vi "Receiver 17 new version.vi"   [LabVIEW 2012]
uses:
  <vilib>/NXT/Block Support/NXT_MessageMailbox.ctl
  <vilib>/NXT/Subs/MotorOutput.ctl
  <vilib>/NXT/Block Support/NXT_InputPort.ctl
  <vilib>/NXT/Dual Mode Library/Waits/Wait_Num.vi
  <vilib>/NXT/Dual Mode Library/BT/BlueTooth_Read_string.vi
  <vilib>/NXT/Dual Mode Library/Display/drawText.vi
types:
  T1 = typedef "LVHSConnector.ctl" = refnum<class "BrickReference.lvclass">
  T2 = typedef "NXT_MessageMailbox.ctl" = u8
  T3 = typedef "MotorOutput.ctl" = u8
  T4 = typedef "NXT_InputPort.ctl" = u32
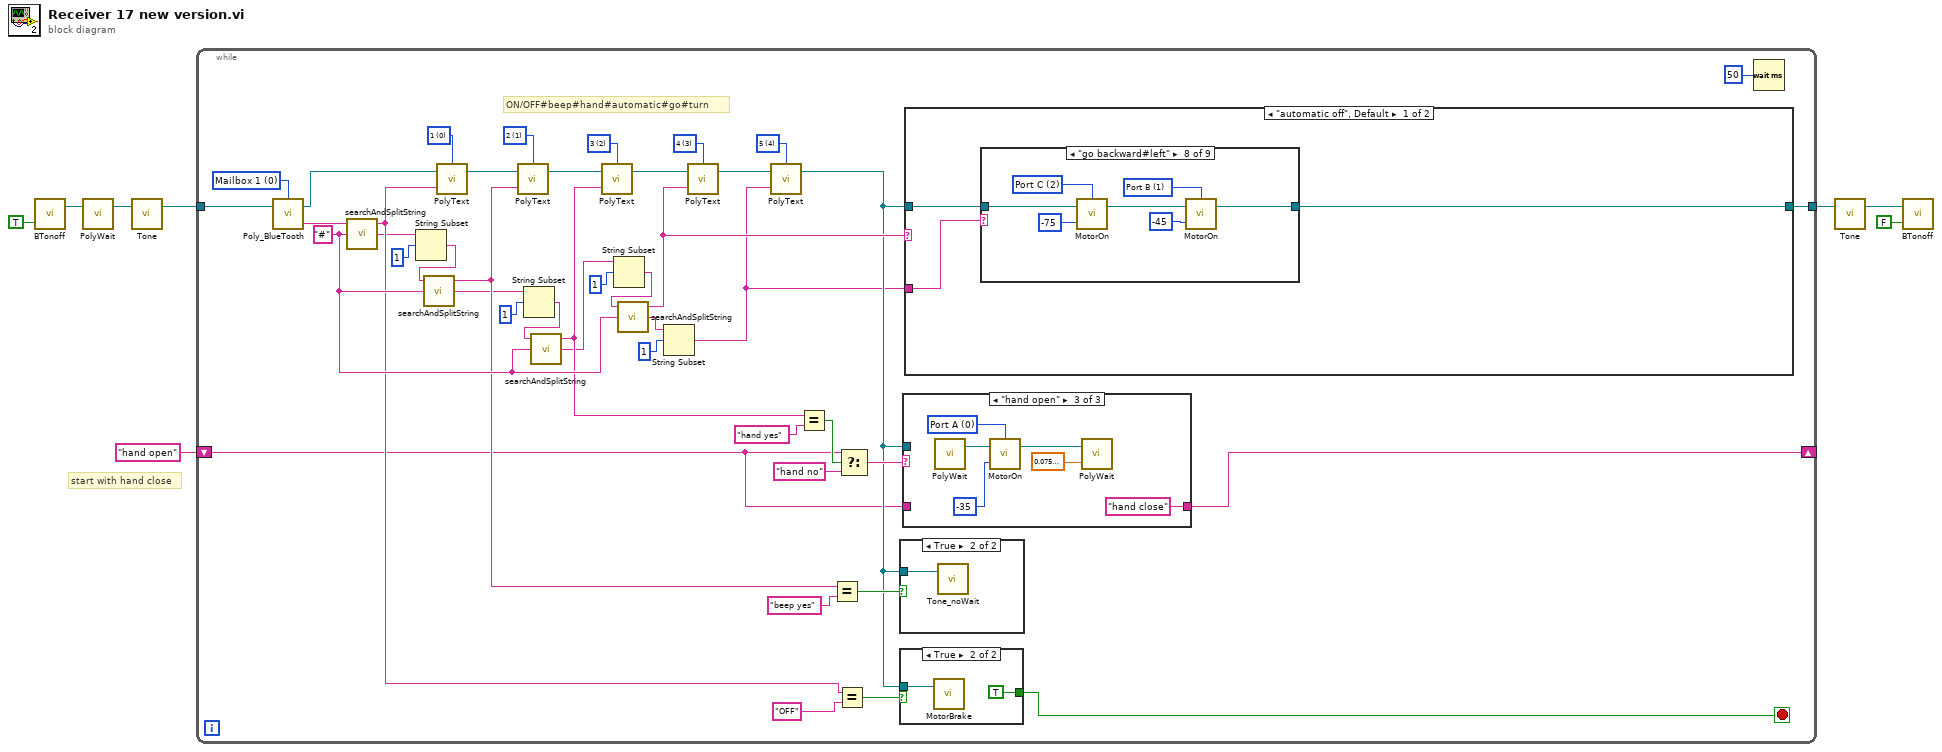
[diagram p0: block diagram]
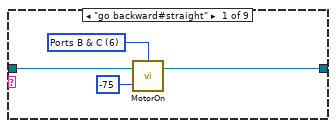
[diagram p2: hidden frame]
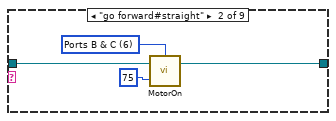
[diagram p3: hidden frame]
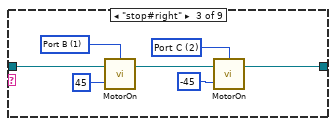
[diagram p4: hidden frame]
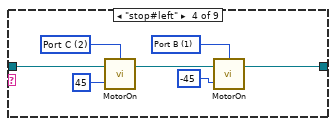
[diagram p5: hidden frame]
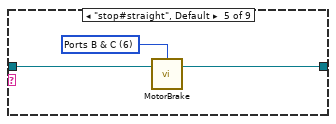
[diagram p6: hidden frame]
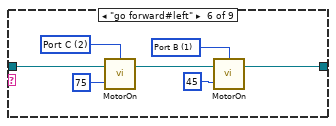
[diagram p7: hidden frame]
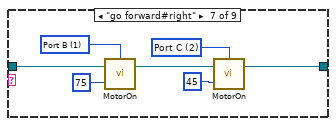
[diagram p8: hidden frame]
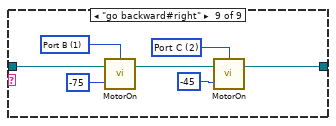
[diagram p9: hidden frame]
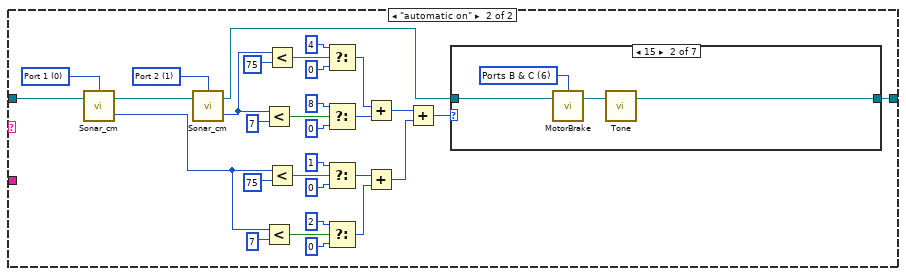
[diagram p10: hidden frame]
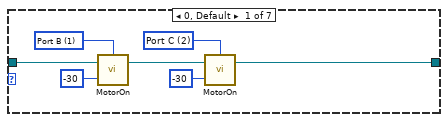
[diagram p11: hidden frame]
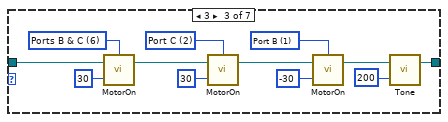
[diagram p12: hidden frame]
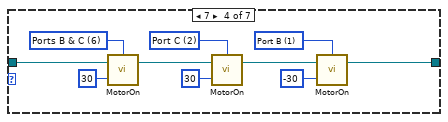
[diagram p13: hidden frame]
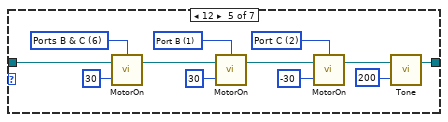
[diagram p14: hidden frame]
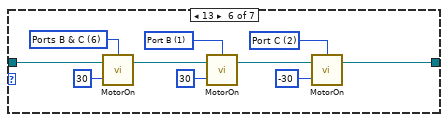
[diagram p15: hidden frame]
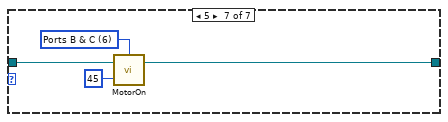
[diagram p16: hidden frame]
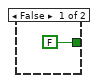
[diagram p17: hidden frame]
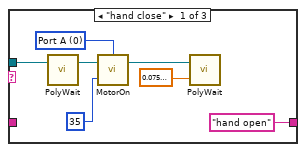
[diagram p19: hidden frame]
diagram:
  # "start with hand close"
  n1 = call <vilib>:"BTonoff.vi"("On/Off"=TRUE) -> ("NXT/EV3"=w6:T1)  [unwired: 2 in, 1 out]
  n2 = call-poly <vilib>:"PolyWait.vi"("NXT/EV3"=w6) -> ("NXT/EV3"=w4:T1)  [unwired: 3 in]
  n3 = call <vilib>:"Tone.vi"("NXT/EV3"=w4) -> ("NXT/EV3"=w3:T1)  [unwired: 3 in]
  n4 = while {
    tunnel: w3 -> [w50]
    shift-right: [w46] -> _
    shift-left: "hand open" -> [w10]
    tunnel: [w41] -> w1
    stop <- w36 stop-if-true
    w28 = i16 4 items=["1", "2", "3", "4", "5", "6", "7", "8", "9", "10", "11", "12"] ("Line")
    w30 = i16 3 items=["1", "2", "3", "4", "5", "6", "7", "8", "9", "10", "11", "12"] ("Line")
    w32 = i16 2 items=["1", "2", "3", "4", "5", "6", "7", "8", "9", "10", "11", "12"] ("Line")
    w34 = i16 1 items=["1", "2", "3", "4", "5", "6", "7", "8", "9", "10", "11", "12"] ("Line")
    w35 = i16 0 items=["1", "2", "3", "4", "5", "6", "7", "8", "9", "10", "11", "12"] ("Line")
    w39 = "#" ("search string/char (-)")
    w52 = T2 0 items=["Mailbox 1", "Mailbox 2", "Mailbox 3", "Mailbox 4", "Mailbox 5", "Mailbox 6", "Mailbox 7", "Mailbox 8", "Mailbox 9", "Mailbox 10"] ("Mailbox")
    # "ON/OFF#beep#hand#automatic#go#turn"
    n5 = call-poly <vilib>:"Poly_BlueTooth.vi"("NXT/EV3"=w50, "Mailbox"=w52) -> ("Message"=w40:string, "NXT/EV3"=w26:T1)  [unwired: 1 in]
    n6 = call <vilib>:"searchAndSplitString.vi"("search string/char (-)"=w39, "string"=w40) -> ("match + rest of string"=w18:string, "substring before match"=w25:string)  [unwired: 1 in, 1 out]
    n7 = String Subset(string=w18, offset (0)=1) -> (substring=w14:string)  [unwired: 1 in]
    n8 = call <vilib>:"searchAndSplitString.vi"("search string/char (-)"=w39, "string"=w14) -> ("match + rest of string"=w16:string, "substring before match"=w24:string)  [unwired: 1 in, 1 out]
    n9 = call-poly <vilib>:"PolyText.vi"("Text"=w25, "NXT/EV3"=w26, "Line"=w35) -> ("NXT/EV3"=w33:T1)  [unwired: 1 in]
    n10 = call-poly <vilib>:"PolyText.vi"("Text"=w24, "NXT/EV3"=w33, "Line"=w34) -> ("NXT/EV3"=w31:T1)  [unwired: 1 in]
    n11 = String Subset(string=w16, offset (0)=1) -> (substring=w15:string)  [unwired: 1 in]
    n12 = call <vilib>:"searchAndSplitString.vi"("search string/char (-)"=w39, "string"=w15) -> ("match + rest of string"=w12:string, "substring before match"=w23:string)  [unwired: 1 in, 1 out]
    n13 = call-poly <vilib>:"PolyText.vi"("Text"=w23, "NXT/EV3"=w31, "Line"=w32) -> ("NXT/EV3"=w29:T1)  [unwired: 1 in]
    n14 = String Subset(string=w12, offset (0)=1) -> (substring=w11:string)  [unwired: 1 in]
    n15 = call <vilib>:"searchAndSplitString.vi"("search string/char (-)"=w39, "string"=w11) -> ("match + rest of string"=w37:string, "substring before match"=w22:string)  [unwired: 1 in, 1 out]
    n16 = String Subset(string=w37, offset (0)=1) -> (substring=w20:string)  [unwired: 1 in]
    n17 = call-poly <vilib>:"PolyText.vi"("Text"=w22, "NXT/EV3"=w29, "Line"=w30) -> ("NXT/EV3"=w27:T1)  [unwired: 1 in]
    n18 = call-poly <vilib>:"PolyText.vi"("Text"=w20, "NXT/EV3"=w27, "Line"=w28) -> ("NXT/EV3"=w21:T1)  [unwired: 1 in]
    n19 = Equal?(x=w23, y="hand yes") -> (x = y?=w48:bool)
    n20 = Equal?(x=w24, y="beep yes") -> (x = y?=w44:bool)
    n21 = Equal?(x=w25, y="OFF") -> (x = y?=w42:bool)
    n22 = Select(t=w10, s=w48, f="hand no") -> (s? t:f=w47:string)
    n23 = case shown="True" w44 {
      tunnel: w21 -> [_ w202]
      frame False {
      }
      frame True {
        n24 = call <vilib>:"Tone_noWait.vi"("NXT/EV3"=w202) -> ()  [unwired: 3 in, 1 out]
      }
    }
    n25 = case shown="True" w42 {
      tunnel: [FALSE TRUE] -> w36
      tunnel: w21 -> [_ w200]
      frame False {
      }
      frame True {
        n26 = call <vilib>:"MotorBrake.vi"("NXT/EV3"=w200) -> ()  [unwired: 3 in, 1 out]
      }
    }
    n27 = case shown="\"hand open\"" w47 {
      tunnel: ["hand open" w210 "hand close"] -> w46
      tunnel: w21 -> [w203 _ _]
      tunnel: w10 -> [_ w210 _]
      frame "hand close" {
        w209 = T3 0 items=["Port A"=0, "Port B"=1, "Port C"=2, "Ports A & B"=4, "Ports A & C"=5, "Ports B & C"=6, "All Ports"=3] ("Output Port (All Ports)")
        n28 = call-poly <vilib>:"PolyWait.vi"("NXT/EV3"=w203) -> ("NXT/EV3"=w205:T1)  [unwired: 3 in]
        n29 = call <vilib>:"MotorOn.vi"("Power (75)"=35, "NXT/EV3"=w205, "Output Port (All Ports)"=w209) -> ("NXT/EV3"=w207:T1)  [unwired: 1 in]
        n30 = call-poly <vilib>:"PolyWait.vi"("Time (1 sec)"=sgl 0.075, "NXT/EV3"=w207) -> ()  [unwired: 2 in, 1 out]
      }
      frame "hand no", Default {
      }
      frame "hand open" {
        w216 = T3 0 items=["Port A"=0, "Port B"=1, "Port C"=2, "Ports A & B"=4, "Ports A & C"=5, "Ports B & C"=6, "All Ports"=3] ("Output Port (All Ports)")
        n31 = call-poly <vilib>:"PolyWait.vi"() -> ("NXT/EV3"=w212:T1)  [unwired: 4 in]
        n32 = call <vilib>:"MotorOn.vi"("Power (75)"=-35, "NXT/EV3"=w212, "Output Port (All Ports)"=w216) -> ("NXT/EV3"=w213:T1)  [unwired: 1 in]
        n33 = call-poly <vilib>:"PolyWait.vi"("Time (1 sec)"=sgl 0.075, "NXT/EV3"=w213) -> ()  [unwired: 2 in, 1 out]
      }
    }
    n34 = case shown="\"automatic off\", Default" w22 {
      tunnel: w21 -> [w55 w110]
      tunnel: [w54 w109] -> w41
      tunnel: w20 -> [w53 _]
      frame "automatic off", Default {
        n35 = case shown="\"go backward#left\"" w53 {
          tunnel: w55 -> [w57 w63 w65 w77 w80 w82 w89 w96 w103]
          tunnel: [w56 w60 w64 w71 w78 w81 w88 w95 w102] -> w54
          frame "go backward#straight" {
            w59 = T3 6 items=["Port A"=0, "Port B"=1, "Port C"=2, "Ports A & B"=4, "Ports A & C"=5, "Ports B & C"=6, "All Ports"=3] ("Output Port (All Ports)")
            n36 = call <vilib>:"MotorOn.vi"("Power (75)"=-75, "NXT/EV3"=w57, "Output Port (All Ports)"=w59) -> ("NXT/EV3"=w56:T1)  [unwired: 1 in]
          }
          frame "go forward#straight" {
            w61 = T3 6 items=["Port A"=0, "Port B"=1, "Port C"=2, "Ports A & B"=4, "Ports A & C"=5, "Ports B & C"=6, "All Ports"=3] ("Output Port (All Ports)")
            n37 = call <vilib>:"MotorOn.vi"("Power (75)"=75, "NXT/EV3"=w63, "Output Port (All Ports)"=w61) -> ("NXT/EV3"=w60:T1)  [unwired: 1 in]
          }
          frame "stop#right" {
            w68 = T3 2 items=["Port A"=0, "Port B"=1, "Port C"=2, "Ports A & B"=4, "Ports A & C"=5, "Ports B & C"=6, "All Ports"=3] ("Output Port (All Ports)")
            w69 = T3 1 items=["Port A"=0, "Port B"=1, "Port C"=2, "Ports A & B"=4, "Ports A & C"=5, "Ports B & C"=6, "All Ports"=3] ("Output Port (All Ports)")
            n38 = call <vilib>:"MotorOn.vi"("Power (75)"=45, "NXT/EV3"=w65, "Output Port (All Ports)"=w69) -> ("NXT/EV3"=w70:T1)  [unwired: 1 in]
            n39 = call <vilib>:"MotorOn.vi"("Power (75)"=-45, "NXT/EV3"=w70, "Output Port (All Ports)"=w68) -> ("NXT/EV3"=w64:T1)  [unwired: 1 in]
          }
          frame "stop#left" {
            w74 = T3 1 items=["Port A"=0, "Port B"=1, "Port C"=2, "Ports A & B"=4, "Ports A & C"=5, "Ports B & C"=6, "All Ports"=3] ("Output Port (All Ports)")
            w75 = T3 2 items=["Port A"=0, "Port B"=1, "Port C"=2, "Ports A & B"=4, "Ports A & C"=5, "Ports B & C"=6, "All Ports"=3] ("Output Port (All Ports)")
            n40 = call <vilib>:"MotorOn.vi"("Power (75)"=45, "NXT/EV3"=w77, "Output Port (All Ports)"=w75) -> ("NXT/EV3"=w76:T1)  [unwired: 1 in]
            n41 = call <vilib>:"MotorOn.vi"("Power (75)"=-45, "NXT/EV3"=w76, "Output Port (All Ports)"=w74) -> ("NXT/EV3"=w71:T1)  [unwired: 1 in]
          }
          frame "stop#straight", Default {
            w79 = T3 6 items=["Port A"=0, "Port B"=1, "Port C"=2, "Ports A & B"=4, "Ports A & C"=5, "Ports B & C"=6, "All Ports"=3] ("Port (All Ports)")
            n42 = call <vilib>:"MotorBrake.vi"("NXT/EV3"=w80, "Port (All Ports)"=w79) -> ("NXT/EV3"=w78:T1)  [unwired: 2 in]
          }
          frame "go forward#left" {
            w85 = T3 1 items=["Port A"=0, "Port B"=1, "Port C"=2, "Ports A & B"=4, "Ports A & C"=5, "Ports B & C"=6, "All Ports"=3] ("Output Port (All Ports)")
            w86 = T3 2 items=["Port A"=0, "Port B"=1, "Port C"=2, "Ports A & B"=4, "Ports A & C"=5, "Ports B & C"=6, "All Ports"=3] ("Output Port (All Ports)")
            n43 = call <vilib>:"MotorOn.vi"("Power (75)"=75, "NXT/EV3"=w82, "Output Port (All Ports)"=w86) -> ("NXT/EV3"=w87:T1)  [unwired: 1 in]
            n44 = call <vilib>:"MotorOn.vi"("Power (75)"=45, "NXT/EV3"=w87, "Output Port (All Ports)"=w85) -> ("NXT/EV3"=w81:T1)  [unwired: 1 in]
          }
          frame "go forward#right" {
            w92 = T3 2 items=["Port A"=0, "Port B"=1, "Port C"=2, "Ports A & B"=4, "Ports A & C"=5, "Ports B & C"=6, "All Ports"=3] ("Output Port (All Ports)")
            w93 = T3 1 items=["Port A"=0, "Port B"=1, "Port C"=2, "Ports A & B"=4, "Ports A & C"=5, "Ports B & C"=6, "All Ports"=3] ("Output Port (All Ports)")
            n45 = call <vilib>:"MotorOn.vi"("Power (75)"=75, "NXT/EV3"=w89, "Output Port (All Ports)"=w93) -> ("NXT/EV3"=w94:T1)  [unwired: 1 in]
            n46 = call <vilib>:"MotorOn.vi"("Power (75)"=45, "NXT/EV3"=w94, "Output Port (All Ports)"=w92) -> ("NXT/EV3"=w88:T1)  [unwired: 1 in]
          }
          frame "go backward#left" {
            w99 = T3 1 items=["Port A"=0, "Port B"=1, "Port C"=2, "Ports A & B"=4, "Ports A & C"=5, "Ports B & C"=6, "All Ports"=3] ("Output Port (All Ports)")
            w100 = T3 2 items=["Port A"=0, "Port B"=1, "Port C"=2, "Ports A & B"=4, "Ports A & C"=5, "Ports B & C"=6, "All Ports"=3] ("Output Port (All Ports)")
            n47 = call <vilib>:"MotorOn.vi"("Power (75)"=-75, "NXT/EV3"=w96, "Output Port (All Ports)"=w100) -> ("NXT/EV3"=w101:T1)  [unwired: 1 in]
            n48 = call <vilib>:"MotorOn.vi"("Power (75)"=-45, "NXT/EV3"=w101, "Output Port (All Ports)"=w99) -> ("NXT/EV3"=w95:T1)  [unwired: 1 in]
          }
          frame "go backward#right" {
            w106 = T3 2 items=["Port A"=0, "Port B"=1, "Port C"=2, "Ports A & B"=4, "Ports A & C"=5, "Ports B & C"=6, "All Ports"=3] ("Output Port (All Ports)")
            w107 = T3 1 items=["Port A"=0, "Port B"=1, "Port C"=2, "Ports A & B"=4, "Ports A & C"=5, "Ports B & C"=6, "All Ports"=3] ("Output Port (All Ports)")
            n49 = call <vilib>:"MotorOn.vi"("Power (75)"=-75, "NXT/EV3"=w103, "Output Port (All Ports)"=w107) -> ("NXT/EV3"=w108:T1)  [unwired: 1 in]
            n50 = call <vilib>:"MotorOn.vi"("Power (75)"=-45, "NXT/EV3"=w108, "Output Port (All Ports)"=w106) -> ("NXT/EV3"=w102:T1)  [unwired: 1 in]
          }
        }
      }
      frame "automatic on" {
        w127 = T4 1 items=["Port 1", "Port 2", "Port 3", "Port 4"] ("Port (Port 4)")
        w139 = T4 0 items=["Port 1", "Port 2", "Port 3", "Port 4"] ("Port (Port 4)")
        n51 = call <vilib>:"Sonar_cm.vi"("NXT/EV3"=w110, "Port (Port 4)"=w139) -> ("Distance (cm)"=w137:i16, "NXT/EV3"=w115:T1)  [unwired: 1 in]
        n52 = call <vilib>:"Sonar_cm.vi"("NXT/EV3"=w115, "Port (Port 4)"=w127) -> ("Distance (cm)"=w125:i16, "NXT/EV3"=w111:T1)  [unwired: 1 in]
        n53 = Less?(x=w125, y=i16 7) -> (x < y?=w124:bool)
        n54 = Less?(x=w137, y=i16 7) -> (x < y?=w136:bool)
        n55 = Less?(x=w125, y=i16 75) -> (x < y?=w126:bool)
        n56 = Less?(x=w137, y=i16 75) -> (x < y?=w138:bool)
        n57 = Select(t=i16 4 ("y"), s=w126, f=i16 0 ("y")) -> (s? t:f=w123:i16)
        n58 = Select(t=i16 8 ("y"), s=w124, f=i16 0 ("y")) -> (s? t:f=w122:i16)
        n59 = Select(t=i16 1 ("y"), s=w138, f=i16 0 ("y")) -> (s? t:f=w135:i16)
        n60 = Select(t=i16 2 ("y"), s=w136, f=i16 0 ("y")) -> (s? t:f=w134:i16)
        n61 = Add(x=w123, y=w122) -> (x+y=w114:i16)
        n62 = Add(x=w135, y=w134) -> (x+y=w113:i16)
        n63 = Add(x=w114, y=w113) -> (x+y=w112:i16)
        n64 = case shown="15" w112 {
          tunnel: w111 -> [w141 w150 w155 w165 w177 w187 w196]
          tunnel: [w140 w147 w151 w163 w173 w185 w195] -> w109
          frame 0, Default {
            w144 = T3 2 items=["Port A"=0, "Port B"=1, "Port C"=2, "Ports A & B"=4, "Ports A & C"=5, "Ports B & C"=6, "All Ports"=3] ("Output Port (All Ports)")
            w145 = T3 1 items=["Port A"=0, "Port B"=1, "Port C"=2, "Ports A & B"=4, "Ports A & C"=5, "Ports B & C"=6, "All Ports"=3] ("Output Port (All Ports)")
            n65 = call <vilib>:"MotorOn.vi"("Power (75)"=-30, "NXT/EV3"=w141, "Output Port (All Ports)"=w145) -> ("NXT/EV3"=w146:T1)  [unwired: 1 in]
            n66 = call <vilib>:"MotorOn.vi"("Power (75)"=-30, "NXT/EV3"=w146, "Output Port (All Ports)"=w144) -> ("NXT/EV3"=w140:T1)  [unwired: 1 in]
          }
          frame 15 {
            w149 = T3 6 items=["Port A"=0, "Port B"=1, "Port C"=2, "Ports A & B"=4, "Ports A & C"=5, "Ports B & C"=6, "All Ports"=3] ("Port (All Ports)")
            n67 = call <vilib>:"MotorBrake.vi"("NXT/EV3"=w150, "Port (All Ports)"=w149) -> ("NXT/EV3"=w148:T1)  [unwired: 2 in]
            n68 = call <vilib>:"Tone.vi"("NXT/EV3"=w148) -> ("NXT/EV3"=w147:T1)  [unwired: 3 in]
          }
          frame 3 {
            w156 = T3 6 items=["Port A"=0, "Port B"=1, "Port C"=2, "Ports A & B"=4, "Ports A & C"=5, "Ports B & C"=6, "All Ports"=3] ("Output Port (All Ports)")
            w161 = T3 1 items=["Port A"=0, "Port B"=1, "Port C"=2, "Ports A & B"=4, "Ports A & C"=5, "Ports B & C"=6, "All Ports"=3] ("Output Port (All Ports)")
            w162 = T3 2 items=["Port A"=0, "Port B"=1, "Port C"=2, "Ports A & B"=4, "Ports A & C"=5, "Ports B & C"=6, "All Ports"=3] ("Output Port (All Ports)")
            n69 = call <vilib>:"MotorOn.vi"("Power (75)"=30, "NXT/EV3"=w155, "Output Port (All Ports)"=w156) -> ("NXT/EV3"=w154:T1)  [unwired: 1 in]
            n70 = call <vilib>:"MotorOn.vi"("Power (75)"=30, "NXT/EV3"=w154, "Output Port (All Ports)"=w162) -> ("NXT/EV3"=w158:T1)  [unwired: 1 in]
            n71 = call <vilib>:"MotorOn.vi"("Power (75)"=-30, "NXT/EV3"=w158, "Output Port (All Ports)"=w161) -> ("NXT/EV3"=w153:T1)  [unwired: 1 in]
            n72 = call <vilib>:"Tone.vi"("Duration (500 ms)"=u16 200, "NXT/EV3"=w153) -> ("NXT/EV3"=w151:T1)  [unwired: 2 in]
          }
          frame 7 {
            w166 = T3 6 items=["Port A"=0, "Port B"=1, "Port C"=2, "Ports A & B"=4, "Ports A & C"=5, "Ports B & C"=6, "All Ports"=3] ("Output Port (All Ports)")
            w171 = T3 1 items=["Port A"=0, "Port B"=1, "Port C"=2, "Ports A & B"=4, "Ports A & C"=5, "Ports B & C"=6, "All Ports"=3] ("Output Port (All Ports)")
            w172 = T3 2 items=["Port A"=0, "Port B"=1, "Port C"=2, "Ports A & B"=4, "Ports A & C"=5, "Ports B & C"=6, "All Ports"=3] ("Output Port (All Ports)")
            n73 = call <vilib>:"MotorOn.vi"("Power (75)"=30, "NXT/EV3"=w165, "Output Port (All Ports)"=w166) -> ("NXT/EV3"=w164:T1)  [unwired: 1 in]
            n74 = call <vilib>:"MotorOn.vi"("Power (75)"=30, "NXT/EV3"=w164, "Output Port (All Ports)"=w172) -> ("NXT/EV3"=w168:T1)  [unwired: 1 in]
            n75 = call <vilib>:"MotorOn.vi"("Power (75)"=-30, "NXT/EV3"=w168, "Output Port (All Ports)"=w171) -> ("NXT/EV3"=w163:T1)  [unwired: 1 in]
          }
          frame 12 {
            w178 = T3 6 items=["Port A"=0, "Port B"=1, "Port C"=2, "Ports A & B"=4, "Ports A & C"=5, "Ports B & C"=6, "All Ports"=3] ("Output Port (All Ports)")
            w181 = T3 2 items=["Port A"=0, "Port B"=1, "Port C"=2, "Ports A & B"=4, "Ports A & C"=5, "Ports B & C"=6, "All Ports"=3] ("Output Port (All Ports)")
            w180 = T3 1 items=["Port A"=0, "Port B"=1, "Port C"=2, "Ports A & B"=4, "Ports A & C"=5, "Ports B & C"=6, "All Ports"=3] ("Output Port (All Ports)")
            n76 = call <vilib>:"MotorOn.vi"("Power (75)"=30, "NXT/EV3"=w177, "Output Port (All Ports)"=w178) -> ("NXT/EV3"=w176:T1)  [unwired: 1 in]
            n77 = call <vilib>:"MotorOn.vi"("Power (75)"=30, "NXT/EV3"=w176, "Output Port (All Ports)"=w180) -> ("NXT/EV3"=w184:T1)  [unwired: 1 in]
            n78 = call <vilib>:"MotorOn.vi"("Power (75)"=-30, "NXT/EV3"=w184, "Output Port (All Ports)"=w181) -> ("NXT/EV3"=w174:T1)  [unwired: 1 in]
            n79 = call <vilib>:"Tone.vi"("Duration (500 ms)"=u16 200, "NXT/EV3"=w174) -> ("NXT/EV3"=w173:T1)  [unwired: 2 in]
          }
          frame 13 {
            w188 = T3 6 items=["Port A"=0, "Port B"=1, "Port C"=2, "Ports A & B"=4, "Ports A & C"=5, "Ports B & C"=6, "All Ports"=3] ("Output Port (All Ports)")
            w191 = T3 2 items=["Port A"=0, "Port B"=1, "Port C"=2, "Ports A & B"=4, "Ports A & C"=5, "Ports B & C"=6, "All Ports"=3] ("Output Port (All Ports)")
            w190 = T3 1 items=["Port A"=0, "Port B"=1, "Port C"=2, "Ports A & B"=4, "Ports A & C"=5, "Ports B & C"=6, "All Ports"=3] ("Output Port (All Ports)")
            n80 = call <vilib>:"MotorOn.vi"("Power (75)"=30, "NXT/EV3"=w187, "Output Port (All Ports)"=w188) -> ("NXT/EV3"=w186:T1)  [unwired: 1 in]
            n81 = call <vilib>:"MotorOn.vi"("Power (75)"=30, "NXT/EV3"=w186, "Output Port (All Ports)"=w190) -> ("NXT/EV3"=w194:T1)  [unwired: 1 in]
            n82 = call <vilib>:"MotorOn.vi"("Power (75)"=-30, "NXT/EV3"=w194, "Output Port (All Ports)"=w191) -> ("NXT/EV3"=w185:T1)  [unwired: 1 in]
          }
          frame 5 {
            w197 = T3 6 items=["Port A"=0, "Port B"=1, "Port C"=2, "Ports A & B"=4, "Ports A & C"=5, "Ports B & C"=6, "All Ports"=3] ("Output Port (All Ports)")
            n83 = call <vilib>:"MotorOn.vi"("Power (75)"=45, "NXT/EV3"=w196, "Output Port (All Ports)"=w197) -> ("NXT/EV3"=w195:T1)  [unwired: 1 in]
          }
        }
      }
    }
    n84 = Wait (ms)(milliseconds to wait=u32 50) -> ()  [unwired: 1 out]
  }
  n85 = call <vilib>:"Tone.vi"("NXT/EV3"=w1) -> ("NXT/EV3"=w5:T1)  [unwired: 3 in]
  n86 = call <vilib>:"BTonoff.vi"("On/Off"=FALSE, "NXT/EV3"=w5) -> ()  [unwired: 1 in, 2 out]
